vi "Init.vi"(8 "error in":errorcluster, 10 "log?":bool, 11 "camera.nit in":refnum<class "camera.lvclass">) -> (0 "error out":errorcluster, 3 "camera.nit out":refnum<class "camera.lvclass">)   [LabVIEW 2020, in "camera.lvclass"]
uses:
  camera.lvclass
  camera.lvclass/camera.ctl
  lib/O-PL.dll
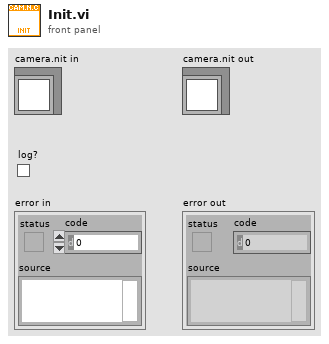
[diagram p1: front panel]
types:
  T1 = typedef "Semaphore RefNum" = refnum<k1>
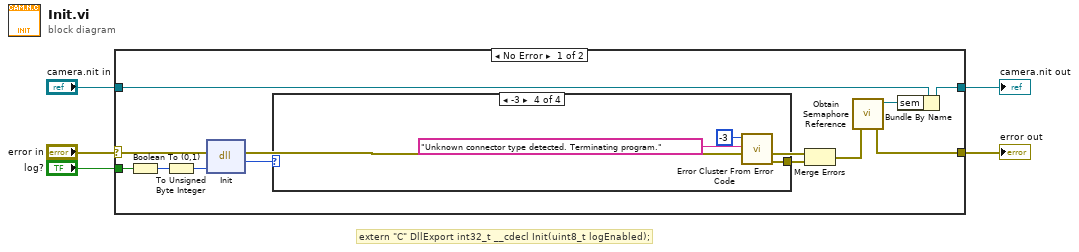
[diagram p0: block diagram]
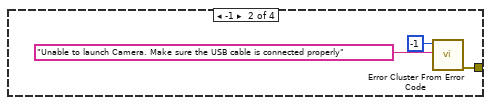
[diagram p3: hidden frame]
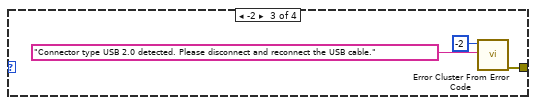
[diagram p4: hidden frame]
diagram:
  # "extern \"C\" DllExport int32_t __cdecl Init(uint8_t logEnabled);"
  n1 = case shown="No Error" "error in" {
    selector: "error in" -> [w17 w28]
    tunnel: [w13 w28] -> w5
    tunnel: "camera.nit in" -> [w16 w27]
    tunnel: [w15 w27] -> w2
    tunnel: "log?" -> [w8 _]
    frame No Error {
      n2 = Boolean To (0,1)(Boolean=w8) -> (0, 1=w7:i16)
      n3 = To Unsigned Byte Integer(number=w7) -> (unsigned 8bit integer=w6:u8)
      n4 = dll-call lib="C:/Users/pittsburger.SOLARIS/Desktop/v0.8/lib/O-PL.dll" fn="Init"(error in=w17, "logEnabled"=w6) -> (error out=w11:errorcluster, "return type"=w12:i32)  [unwired: 3 in, 1 out]
      n5 = case shown="-3" w12 {
        tunnel: [_ w18 w21 w24] -> w10
        frame Default {
        }
        frame -1 {
          n6 = call <vilib>:"Error Cluster From Error Code.vi"("error message (\"\")"="Unable to launch Camera. Make sure the USB cable is connected properly" ("error message"), "error code (0)"=-1) -> ("error out"=w18:errorcluster)  [unwired: 7 in]
        }
        frame -2 {
          n7 = call <vilib>:"Error Cluster From Error Code.vi"("error message (\"\")"="Connector type USB 2.0 detected. Please disconnect and reconnect the USB cable." ("error message"), "error code (0)"=-2) -> ("error out"=w21:errorcluster)  [unwired: 7 in]
        }
        frame -3 {
          n8 = call <vilib>:"Error Cluster From Error Code.vi"("error message (\"\")"="Unknown connector type detected. Terminating program." ("error message"), "error code (0)"=-3) -> ("error out"=w24:errorcluster)  [unwired: 7 in]
        }
      }
      n9 = Merge Errors(w11, w10) -> (w9:errorcluster)
      n10 = call <vilib>:"Obtain Semaphore Reference.vi"("error in (no error)"=w9) -> ("error out"=w13:errorcluster, "semaphore"=w14:T1)  [unwired: 4 in, 1 out]
      n11 = Bundle By Name(cluster=w16, "sem"=w14) -> (w15:refnum<class "camera.lvclass">)
    }
    frame Error {
    }
  }
  "error out" <- w5
  "camera.nit out" <- w2
